vi "Image Sources.vi"() -> ()   [LabVIEW 2020]
uses:
  LabVIEW/g_ar_toolkit.image/ARGB Colour.ctl
  LabVIEW/g_ar_toolkit.common/Image Size (Integer).ctl
  LabVIEW/g_ar_toolkit.image/NewImageARGB.vi
  LabVIEW/g_ar_toolkit.image/NewImageARGB.vi/3321fa97-f432-4e1e-8db9-a0df79aed21b.vi
  LabVIEW/g_ar_toolkit.image/ARGB Colour to U32 Pixel Value.vi
  LabVIEW/g_ar_toolkit.image/ReadImageFileARGB.vi/2358f293-6357-4b7a-bec3-c4e4d03be6e5.vi
  LabVIEW/g_ar_toolkit.common/Module Path.vi
  <vilib>/Utility/error.llb/Error Cluster From Error Code.vi
  LabVIEW/g_ar_toolkit.image/NewImageARGBArray.vi
  LabVIEW/g_ar_toolkit.image/CopyArrayToImagePixels.vi
  LabVIEW/g_ar_toolkit.image/ReadImageFileARGB.vi
  LabVIEW/g_ar_toolkit.image/g_ar_toolkit.image.lvlib
  LabVIEW/g_ar_toolkit.common/g_ar_toolkit.common.lvlib
  LabVIEW/g_ar_toolkit.image/ARGB Image.ctl
  LabVIEW/g_ar_toolkit.image/Greyscale Image.ctl
  LabVIEW/g_ar_toolkit.image/CopyImageGreyscaleMaskARGB.vi
  LabVIEW/g_ar_toolkit.image/ARGBImageSize.vi
  LabVIEW/g_ar_toolkit.image/CopyPixmapToImageFlattenMaskARGB.vi
panel:
  out "3D Picture":refnum<vi>(3d-picture)
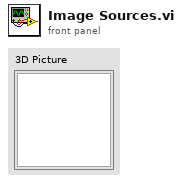
[diagram p1: front panel]
types:
  T1 = typedef "g_ar_toolkit.image.lvlib/Greyscale Image.ctl" = refnum<data-value>
  T2 = typedef "g_ar_toolkit.common.lvlib/Image Size (Integer).ctl" = cluster{"Width":u16, "Height":u16}
  T3 = typedef "g_ar_toolkit.image.lvlib/ARGB Colour.ctl" = cluster{"Alpha":u8, "RGB":u32}
  T4 = typedef "g_ar_toolkit.image.lvlib/ARGB Image.ctl" = refnum<data-value>
  T5 = typedef "imagedata.ctl" = cluster{"image type":i32, "image depth":i32, "image":u8[], "mask":u8[], "colors":u32[], "Rectangle":cluster{"left":i16, "top":i16, "right":i16, "bottom":i16}}
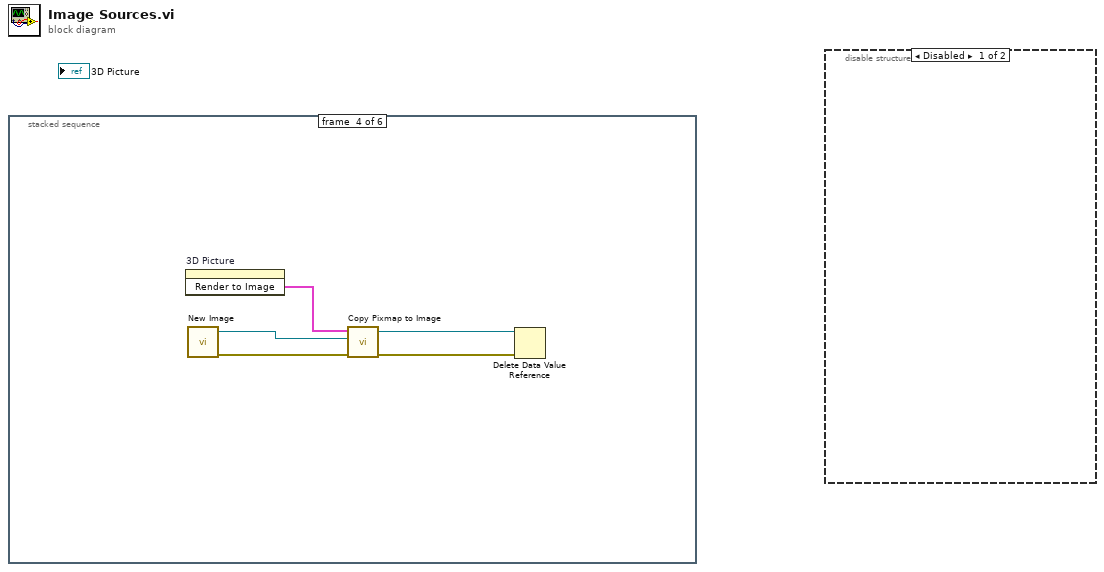
[diagram p0: block diagram]
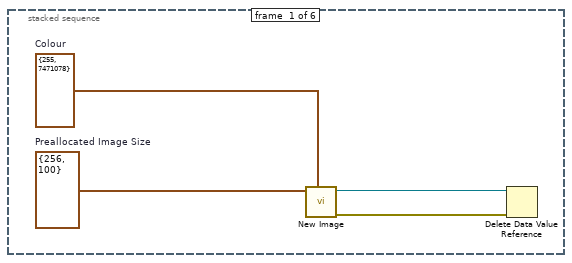
[diagram p3: hidden frame]
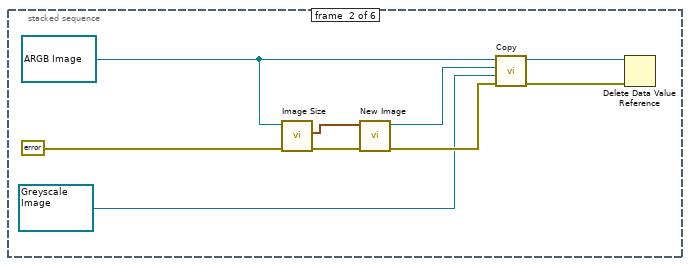
[diagram p4: hidden frame]
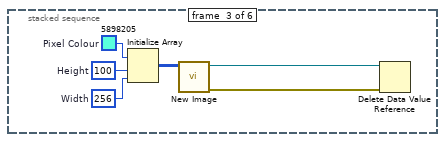
[diagram p5: hidden frame]
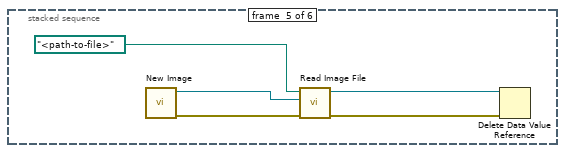
[diagram p6: hidden frame]
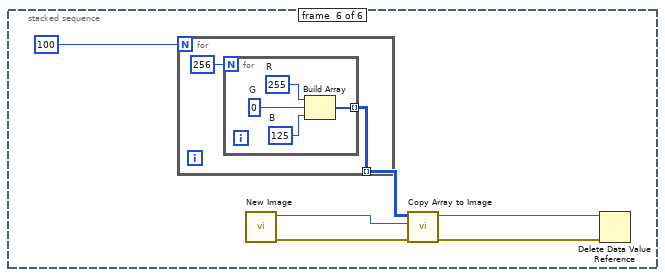
[diagram p7: hidden frame]
diagram:
  n1 = stacked-sequence {
    frame #0 {
      w3 = T2 {"Width"=256, "Height"=100}  # Preallocated Image Size
      w4 = T3 {"Alpha"=255, "RGB"=7471078}  # Colour
      n2 = call-poly "New Image.vi"("Colour (Default: Black)"=w4, "Preallocated Image Size (Default: 0,0)"=w3) -> ("error out"=w1:errorcluster, "New ARGB Image"=w2:T4)  [unwired: 8 in]
      n3 = Delete Data Value Reference(data value reference=w2, error in=w1) -> ()  [unwired: 2 out]
    }
    frame #1 {
      w5 = T4 refnum ("ARGB Image Source")
      n4 = call-poly "Image Size.vi"("error in (no error)"=errorcluster {"status"=FALSE, "code"=0, "source"=""}, "ARGB Image"=w5) -> ("error out"=w7:errorcluster, "Image Size"=w6:T2)  [unwired: 7 in, 1 out]
      n5 = call-poly "New Image.vi"("error in (no error)"=w7, "Preallocated Image Size (Default: 0,0)"=w6) -> ("error out"=w12:errorcluster, "New ARGB Image"=w13:T4)  [unwired: 8 in]
      n6 = call-poly "Copy.vi"("error in (no error)"=w12, "Greyscale Image Mask"=T1 refnum, "ARGB Image Destination"=w13, "ARGB Image Source"=w5) -> ("error out"=w9:errorcluster, "ARGB Image Destination (duplicate)"=w11:T4)  [unwired: 6 in]
      n7 = Delete Data Value Reference(data value reference=w11, error in=w9) -> ()  [unwired: 2 out]
    }
    frame #2 {
      w15 = u32 5898205  # Pixel Colour
      w16 = 256  # Width
      w17 = 100  # Height
      n8 = Initialize Array(w15, w17, w16) -> (w14:u32[][])
      n9 = call-poly "New Image.vi"("U32 ARBG Data  (Default: Empty)"=w14) -> ("error out"=w18:errorcluster, "New ARGB Image"=w19:T4)  [unwired: 9 in]
      n10 = Delete Data Value Reference(data value reference=w19, error in=w18) -> ()  [unwired: 2 out]
    }
    frame #3 {
      n11 = invoke on="3D Picture" class="SceneGraphDisp (strict)" method="Render to Image"() -> ("Get Image"=w20:T5)  [unwired: 3 in, 2 out]
      n12 = call-poly "New Image.vi"() -> ("error out"=w24:errorcluster, "New ARGB Image"=w23:T4)  [unwired: 10 in]
      n13 = call-poly "Copy Pixmap to Image.vi"("error in (no error)"=w24, "ARGB Image Destination"=w23, "Pixmap Image Data"=w20) -> ("error out"=w22:errorcluster, "ARGB Image Destination (duplicate)"=w21:T4)  [unwired: 7 in]
      n14 = Delete Data Value Reference(data value reference=w21, error in=w22) -> ()  [unwired: 2 out]
    }
    frame #4 {
      n15 = call-poly "New Image.vi"() -> ("error out"=w27:errorcluster, "New ARGB Image"=w28:T4)  [unwired: 10 in]
      n16 = call-poly "Read Image File.vi"("error in (no error)"=w27, "ARGB Image Destination"=w28, "Filepath"=path "<path-to-file>") -> ("error out"=w25:errorcluster, "ARGB Image Destination (duplicate)"=w26:T4)  [unwired: 7 in]
      n17 = Delete Data Value Reference(data value reference=w26, error in=w25) -> ()  [unwired: 2 out]
    }
    frame #5 {
      n18 = for {
        N: 100 -> [_]
        tunnel: [w36] -> w31 mode=indexing
        n19 = for {
          N: 256 -> [_]
          tunnel: [w41] -> w36 mode=indexing
          w38 = u8 125  # B
          w39 = u8 0  # G
          w40 = u8 255  # R
          n20 = Build Array(w40, w39, w38) -> (w41:u8[])
        }
      }
      n21 = call-poly "New Image.vi"() -> ("error out"=w34:errorcluster, "New ARGB Image"=w35:T4)  [unwired: 10 in]
      n22 = call-poly "Copy Array to Image.vi"("error in (no error)"=w34, "ARGB Image Destination"=w35, "(A)RGB Pixels Data"=w31) -> ("error out"=w33:errorcluster, "ARGB Image Destination (Duplicate)"=w30:T4)  [unwired: 7 in]
      n23 = Delete Data Value Reference(data value reference=w30, error in=w33) -> ()  [unwired: 2 out]
    }
  }
  n24 = disable-structure shown="Disabled" {
    frame Disabled {
    }
    frame Enabled {
    }
  }
